vi "Main.vi"() -> ()   [LabVIEW 2020]
doc: "Ce VI modèle est conçu pour le modèle de conception Gestionnaire de messages dans une file d'attente.\n\nLa boucle de gestion d'événements génère des messages en fonction des actions sur l'interface utilisateur.\n\nLa boucle de gestion de messages traite les messages générés par la boucle de gestion d'événements ou par d'autres messages. Les messages sont des valeurs chaîne ; il est donc facile d'ajouter de nouveaux messages à la structure condition Conditions de messages de la boucle de gestion de messages Chaque cluster Message peut en outre fournir une valeur optionnelle pour Données de message, un variant qui peut être converti aux données requises pour un message spécifique."
uses:
  controls/UI Data.ctl
  support/Message Queue/Enqueue Message (Single).vi
  <vilib>/Utility/error.llb/Error Cluster From Error Code.vi
  <vilib>/ErrorRing/Error Ring.xnode
  support/Message Queue/Message Queue.lvlib
  support/User Event - Stop/User Event - Stop.lvlib
panel:
  out "Affichage <À remplacer>":string
  in  "Faire action 2 <À remplacer>":bool
  in  "Faire action 1 <À remplacer>":bool
  in  "Quitter":bool
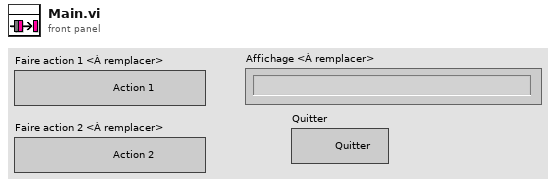
[diagram p1: front panel]
types:
  T1 = typedef "UI Data.ctl" = cluster{"Booléen <À remplacer>":bool, "Chaîne <À remplacer>":string, "Numérique <À remplacer>":dbl, "Réf. Action 1":refnum<vi>, "Réf. Action 2":refnum<vi>, "Réf. Affichage des données":refnum<vi>, "Réf du bouton Quitter":refnum<vi>}
  T2 = cluster{"état":bool, "code":i32, "source":string}
  T3 = typedef "Message Queue.lvlib/All Message Queues.ctl" = cluster{"IU":refnum<queue>}
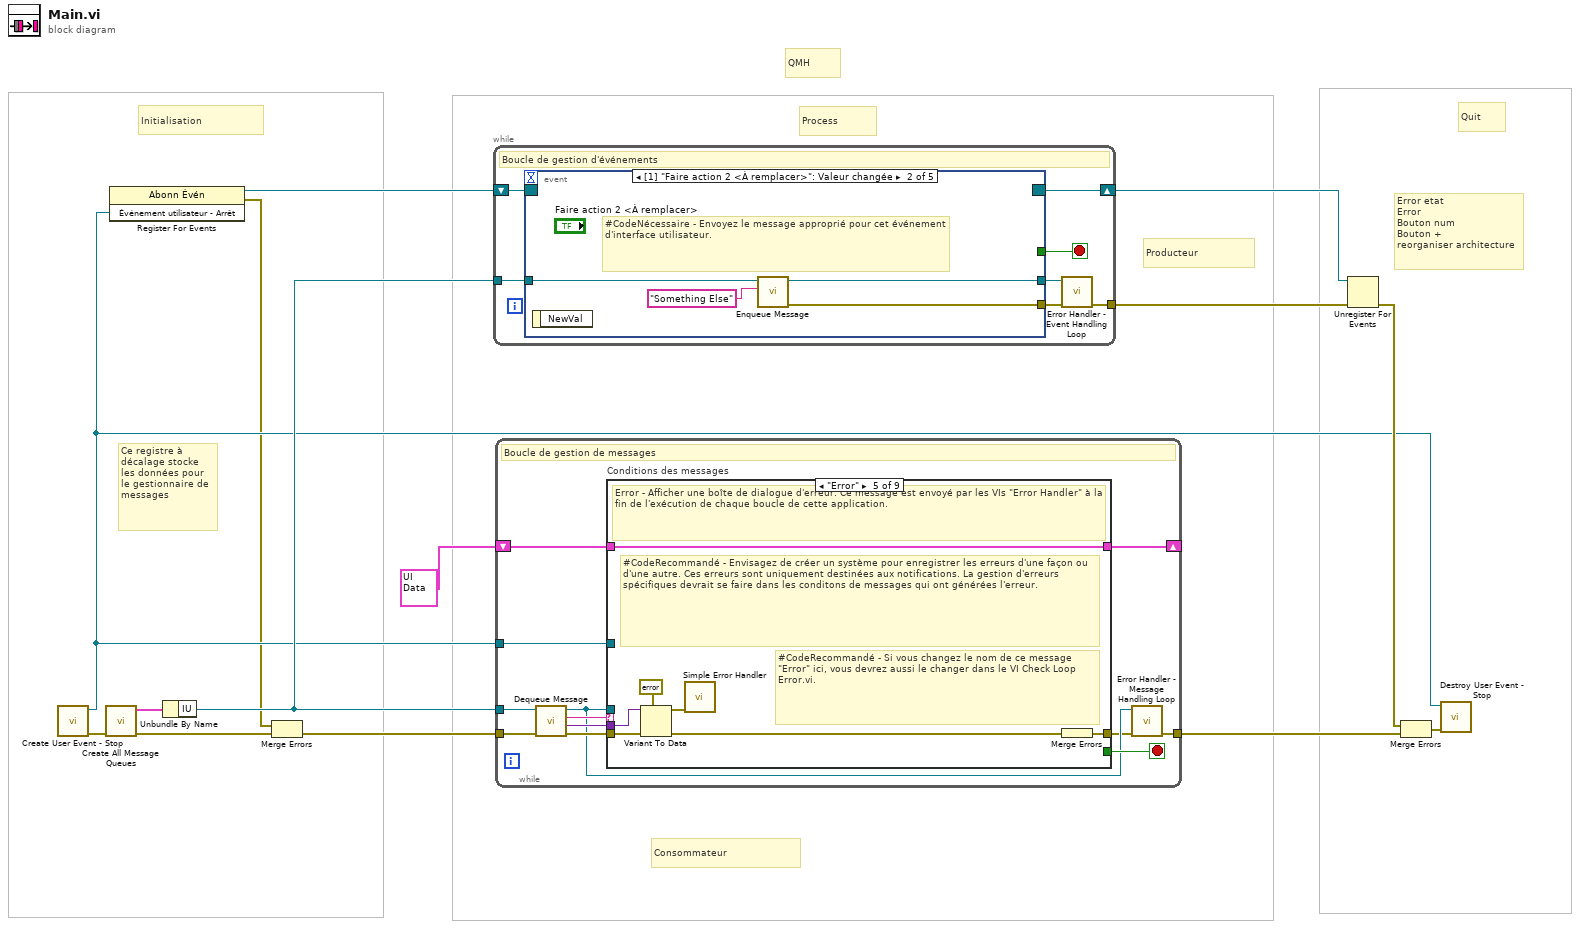
[diagram p0: block diagram]
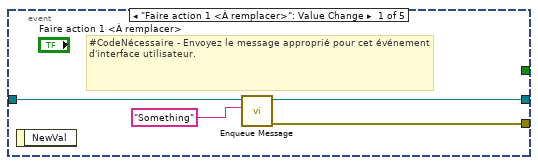
[diagram p2: hidden frame]
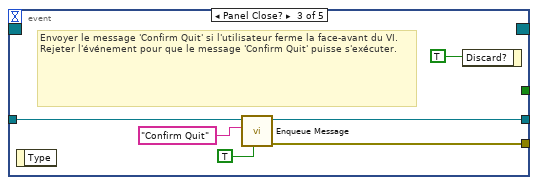
[diagram p3: hidden frame]
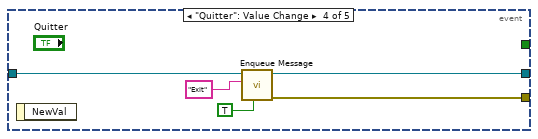
[diagram p4: hidden frame]
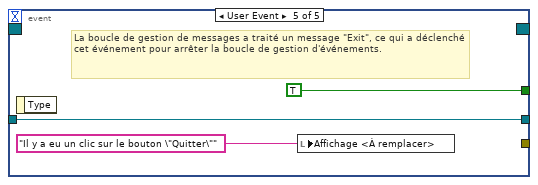
[diagram p5: hidden frame]
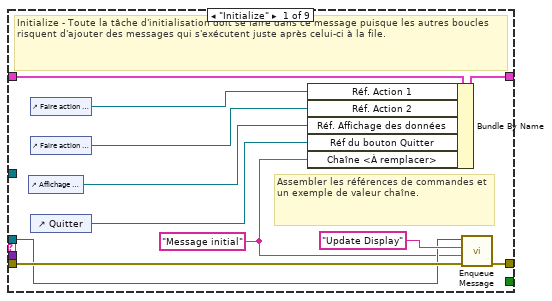
[diagram p6: hidden frame]
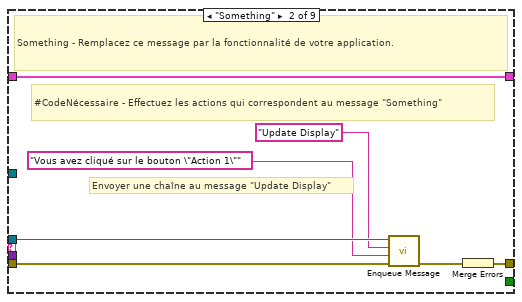
[diagram p7: hidden frame]
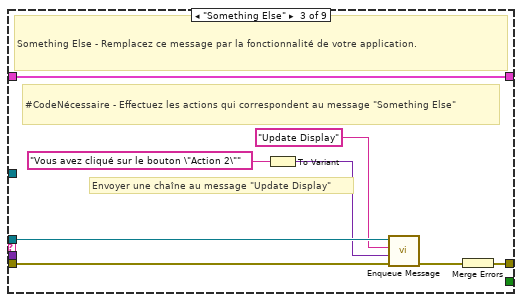
[diagram p8: hidden frame]
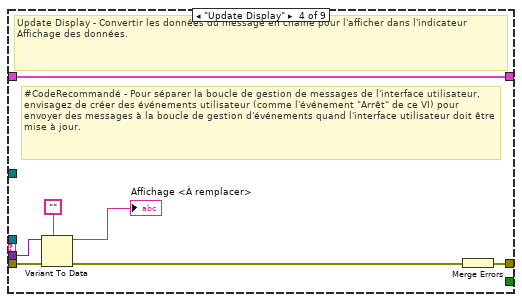
[diagram p9: hidden frame]
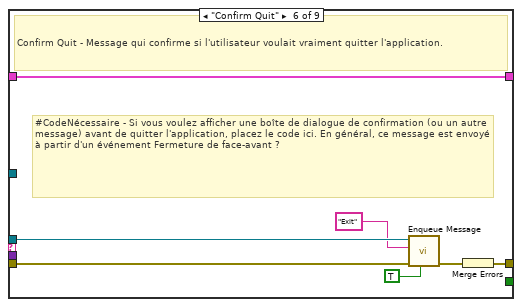
[diagram p10: hidden frame]
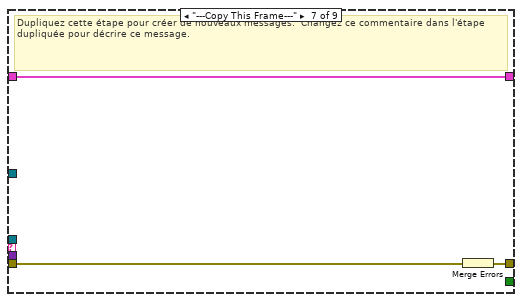
[diagram p11: hidden frame]
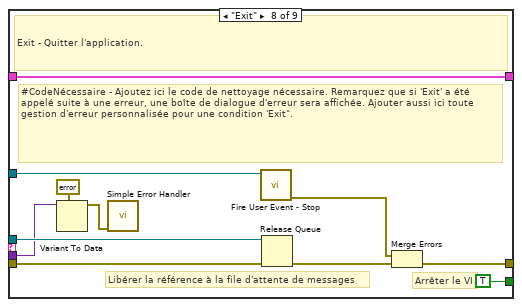
[diagram p12: hidden frame]
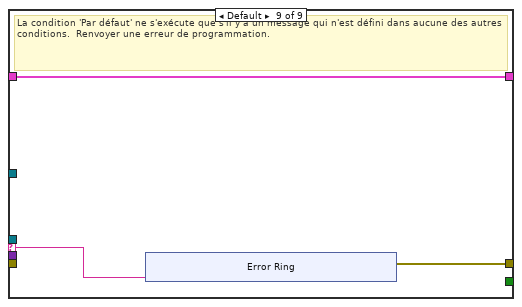
[diagram p13: hidden frame]
diagram:
  # "Error etat\nError\nBouton num\nBouton +\nreorganiser architecture"
  # "QMH"
  # "Consommateur"
  # "Producteur"
  # "Quit"
  # "Process"
  # "Initialisation"
  # "Ce registre à décalage stocke les données pour le gestionnaire de messages"
  n1 = call "Create User Event - Stop.vi"() -> ("error out"=w10:T2, "Événement utilisateur - Arrêt"=w3:refnum<user-event>)  [unwired: 10 in]
  n2 = call "Create All Message Queues.vi"("error in (no error)"=w10) -> ("error out"=w14:T2, "Files d'attente de messages en sortie"=w13:T3)  [unwired: 9 in]
  n3 = register-events(w3) -> (reference out=w4:refnum<event-registration>, error out=w1:errorcluster)  [unwired: 2 in]
  n4 = Unbundle By Name(w13) -> ("IU"=w11:refnum<queue>)
  n5 = Merge Errors(w1, w14) -> (w2:errorcluster)
  n6 = while {
    tunnel: w11 -> [w21]
    shift-right: [w19] -> w7
    shift-left: w4 -> [w20]
    tunnel: [w15] -> w5
    stop <- w17 stop-if-true
    # "Boucle de gestion d'événements"
    n7 = event shown="[1] \"Faire action 2 <À remplacer>\": Valeur changée" {
      selector: w20 -> [_ _ _ _ _]
      dyn-events: [_ _ _ _ _] -> w19
      timeout: _ -> [_ _ _ _ _]
      tunnel: [_ _ _ _ TRUE ("Discard?")] -> w17
      tunnel: w21 -> [w25 w29 w34 w40 w43]
      tunnel: [w22 w26 w33 w39 _] -> w18
      tunnel: [w24 w28 w32 w38 w43] -> w16
      event "Faire action 1 <À remplacer>": Value Change {
        # "#CodeNécessaire - Envoyez le message approprié pour cet événement d'interface utilisateur."
        n8 = event-data() -> ()  [unwired: 1 in, 1 out]
        n9 = call-poly "Enqueue Message.vi"("Message"="Something", "File d'attente de messages"=w25) -> ("error out"=w22:T2, "File d'attente de message dup."=w24:refnum<queue>)  [unwired: 8 in]
      }
      event "Faire action 2 <À remplacer>": Value Change {
        # "#CodeNécessaire - Envoyez le message approprié pour cet événement d'interface utilisateur."
        n10 = event-data() -> ()  [unwired: 1 in, 1 out]
        n11 = call-poly "Enqueue Message.vi"("Message"="Something Else", "File d'attente de messages"=w29) -> ("error out"=w26:T2, "File d'attente de message dup."=w28:refnum<queue>)  [unwired: 8 in]
      }
      event Panel Close? {
        # "Envoyer le message 'Confirm Quit' si l'utilisateur ferme la face-avant du VI. Rejeter l'événement pour que le message 'Confirm Quit' puisse s'exécuter."
        n12 = event-data() -> ()  [unwired: 1 in, 1 out]
        n13 = call-poly "Enqueue Message.vi"("Message prioritaire ? (F)"=TRUE ("Priority Message? (F)"), "Message"="Confirm Quit", "File d'attente de messages"=w34) -> ("error out"=w33:T2, "File d'attente de message dup."=w32:refnum<queue>)  [unwired: 7 in]
        n14 = event-data ("Event Filter Node")("Discard?"=TRUE) -> ()  [unwired: 1 in, 1 out]
      }
      event "Quitter": Value Change {
        n15 = event-data() -> ()  [unwired: 1 in, 1 out]
        n16 = call-poly "Enqueue Message.vi"("Message prioritaire ? (F)"=TRUE ("Priority Message? (F)"), "Message"="Exit", "File d'attente de messages"=w40) -> ("error out"=w39:T2, "File d'attente de message dup."=w38:refnum<queue>)  [unwired: 7 in]
      }
      event User Event {
        # "La boucle de gestion de messages a traité un message \"Exit\", ce qui a déclenché cet événement pour arrêter la boucle de gestion d'événements."
        n17 = event-data() -> ()  [unwired: 1 in, 1 out]
        n18 = local write "Affichage <À remplacer>"("Il y a eu un clic sur le bouton \"Quitter\"" ("VI Stopped")) -> ()
      }
    }
    n19 = call "Error Handler - Event Handling Loop.vi"("error in (no error)"=w18, "File d'attente de messages"=w16) -> ("erreur en entrée dup."=w15:T2)  [unwired: 8 in, 1 out]
  }
  n20 = while {
    tunnel: w11 -> [w47]
    shift-right: [w54] -> _
    shift-left: T1 {"Booléen <À remplacer>"=FALSE, "Chaîne <À remplacer>"="", "Numérique <À remplacer>"=0.0, "Réf. Action 1"=refnum, "Réf. Action 2"=refnum, "Réf. Affichage des données"=refnum, "Réf du bouton Quitter"=refnum} ("Data Cluster") -> [w55]
    tunnel: w3 -> [w52]
    tunnel: w2 -> [w51]
    tunnel: [w45] -> w12
    stop <- w53 stop-if-true
    # "Boucle de gestion de messages"
    n21 = call "Dequeue Message.vi"("error in (no error)"=w51, "File d'attente de messages"=w47) -> ("error out"=w50:T2, "Données de message"=w48:variant, "Message"=w49:string, "File d'attente de message dup."=w46:refnum<queue>)  [unwired: 6 in]
    n22 = case "Conditions des messages" shown="\"Error\"" w49 {
      selector: w49 -> [_ _ _ _ _ _ _ _ w117]
      tunnel: w46 -> [w57 w69 w77 _ _ w98 _ w116 _]
      tunnel: w50 -> [w65 w71 w79 w86 w95 w102 w105 w109 _]
      tunnel: [w66 w72 w80 w87 w89 w100 w103 w112 w118] -> w44
      tunnel: w55 -> [w64 w73 w81 w88 w94 w101 w104 w115 w119]
      tunnel: [w63 w73 w81 w88 w94 w101 w104 w115 w119] -> w54
      tunnel: [_ _ _ _ _ _ _ TRUE _] -> w53
      tunnel: w48 -> [_ _ _ w85 w93 _ _ w106 _]
      tunnel: w52 -> [_ _ _ _ _ _ _ w111 _]
      frame "Initialize" {
        w56 = "Message initial" ("Initial Message")
        # "Assembler les références de commandes et un exemple de valeur chaîne."
        # "Initialize - Toute la tâche d'initialisation doit se faire dans ce message puisque les autres boucles risquent d'ajouter des messages qui s'exécutent juste après celui-ci à la file."
        n23 = control-ref of="Affichage <À remplacer>"() -> (w60:refnum<vi>)
        n24 = control-ref of="Faire action 1 <À remplacer>"() -> (w62:refnum<vi>)
        n25 = control-ref of="Faire action 2 <À remplacer>"() -> (w61:refnum<vi>)
        n26 = control-ref of="Quitter"() -> (w59:refnum<vi>)
        n27 = Bundle By Name(cluster=w64, "Réf. Action 1"=w62, "Réf. Action 2"=w61, "Réf. Affichage des données"=w60, "Réf du bouton Quitter"=w59, "Chaîne <À remplacer>"=w56) -> (w63:T1)
        n28 = call-poly "Enqueue Message.vi"("error in (no error)"=w65, "Données de message"=w56, "Message"="Update Display", "File d'attente de messages"=w57) -> ("error out"=w66:T2)  [unwired: 6 in, 1 out]
      }
      frame "Something" {
        # "Envoyer une chaîne au message \"Update Display\""
        # "#CodeNécessaire - Effectuez les actions qui correspondent au message \"Something\""
        # "Something - Remplacez ce message par la fonctionnalité de votre application."
        n29 = call-poly "Enqueue Message.vi"("error in (no error)"=w71, "Données de message"="Vous avez cliqué sur le bouton \"Action 1\"" ("\"Do Something\" button pressed"), "Message"="Update Display", "File d'attente de messages"=w69) -> ("error out"=w70:T2)  [unwired: 6 in, 1 out]
        n30 = Merge Errors(w70) -> (w72:errorcluster)
      }
      frame "Something Else" {
        # "Envoyer une chaîne au message \"Update Display\""
        # "#CodeNécessaire - Effectuez les actions qui correspondent au message \"Something Else\""
        # "Something Else - Remplacez ce message par la fonctionnalité de votre application."
        n31 = To Variant(anything="Vous avez cliqué sur le bouton \"Action 2\"" ("\"Do Something Else\" button pressed")) -> (Variant=w74:variant)
        n32 = call-poly "Enqueue Message.vi"("error in (no error)"=w79, "Données de message"=w74, "Message"="Update Display", "File d'attente de messages"=w77) -> ("error out"=w78:T2)  [unwired: 6 in, 1 out]
        n33 = Merge Errors(w78) -> (w80:errorcluster)
      }
      frame "Update Display" {
        # "#CodeRecommandé - Pour séparer la boucle de gestion de messages de l'interface utilisateur, envisagez de créer des événements utilisateur (comme l'événement \"Arrêt\" de ce VI) pour envoyer des messages à la boucle de gestion d'événements quand l'interface utilisateur doit être mise à jour."
        # "Update Display - Convertir les données du message en chaîne pour l'afficher dans l'indicateur Affichage des données."
        n34 = Variant To Data(error in=w86, type="", Variant=w85) -> (data=→"Affichage <À remplacer>":string, error out=w83:errorcluster)
        n35 = Merge Errors(w83) -> (w87:errorcluster)
      }
      frame "Error" {
        # "#CodeRecommandé - Si vous changez le nom de ce message \"Error\" ici, vous devrez aussi le changer dans le VI Check Loop Error.vi."
        # "#CodeRecommandé - Envisagez de créer un système pour enregistrer les erreurs d'une façon ou d'une autre. Ces erreurs sont uniquement destinées aux notifications. La gestion d'erreurs spécifiques devrait se faire dans les conditons de messages qui ont générées l'erreur."
        # "Error - Afficher une boîte de dialogue d'erreur. Ce message est envoyé par les VIs \"Error Handler\" à la fin de l'exécution de chaque boucle de cette application."
        n36 = Variant To Data(error in=w95, type=errorcluster {"status"=FALSE, "code"=0, "source"=""} ("error constant"), Variant=w93) -> (data=w91:errorcluster, error out=w90:errorcluster)
        n37 = call <vilib>:"Simple Error Handler.vi"("error in (no error)"=w91) -> ()  [unwired: 4 in, 5 out]
        n38 = Merge Errors(w90) -> (w89:errorcluster)
      }
      frame "Confirm Quit" {
        # "#CodeNécessaire - Si vous voulez afficher une boîte de dialogue de confirmation (ou un autre message) avant de quitter l'application, placez le code ici. En général, ce message est envoyé à partir d'un événement Fermeture de face-avant ?"
        # "Confirm Quit - Message qui confirme si l'utilisateur voulait vraiment quitter l'application."
        n39 = call-poly "Enqueue Message.vi"("Message prioritaire ? (F)"=TRUE ("Priority Message? (F)"), "error in (no error)"=w102, "Message"="Exit", "File d'attente de messages"=w98) -> ("error out"=w99:T2)  [unwired: 6 in, 1 out]
        n40 = Merge Errors(w99) -> (w100:errorcluster)
      }
      frame "---Copy This Frame---" {
        # "Dupliquez cette étape pour créer de nouveaux messages.  Changez ce commentaire dans l'étape dupliquée pour décrire ce message."
        n41 = Merge Errors(w105) -> (w103:errorcluster)
      }
      frame "Exit" {
        # "Arrêter le VI"
        # "Libérer la référence à la file d'attente de messages"
        # "#CodeNécessaire - Ajoutez ici le code de nettoyage nécessaire. Remarquez que si 'Exit' a été appelé suite à une erreur, une boîte de dialogue d'erreur sera affichée. Ajouter aussi ici toute gestion d'erreur personnalisée pour une condition 'Exit\"."
        # "Exit - Quitter l'application."
        n42 = Variant To Data(type=errorcluster {"status"=FALSE, "code"=0, "source"=""} ("error constant"), Variant=w106) -> (data=w107:errorcluster)  [unwired: 1 in, 1 out]
        n43 = call <vilib>:"Simple Error Handler.vi"("error in (no error)"=w107) -> ()  [unwired: 4 in, 5 out]
        n44 = call "Fire User Event - Stop.vi"("Événement utilisateur - Arrêt"=w111) -> ("error out"=w110:T2)  [unwired: 10 in]
        n45 = Release Queue(queue=w116, error in (no error)=w109) -> (error out=w113:errorcluster)  [unwired: 1 in, 2 out]
        n46 = Merge Errors(w110, w113) -> (w112:errorcluster)
      }
      frame Default {
        # "La condition 'Par défaut' ne s'exécute que s'il y a un message qui n'est défini dans aucune des autres conditions.  Renvoyer une erreur de programmation."
        n47 = xnode ("Error Ring")("paramètre 0"=w117) -> ("sortie d'erreur"=w118:errorcluster)
      }
    }
    n48 = call "Error Handler - Message Handling Loop.vi"("error in (no error)"=w44, "File d'attente de messages"=w46) -> ("erreur en entrée dup."=w45:T2)  [unwired: 8 in, 1 out]
  }
  n49 = Unregister For Events(event registration refnum=w7, error in=w5) -> (error out=w8:errorcluster)
  n50 = Merge Errors(w8, w12) -> (w9:errorcluster)
  n51 = call "Destroy User Event - Stop.vi"("error in (no error)"=w9, "Événement utilisateur - Arrêt"=w3) -> ()  [unwired: 9 in, 1 out]
